vi "generate_smgr.vi"() -> ()   [LabVIEW 2010]
uses:
  lib/Global 2.vi
  <vilib>/measure/NI_MABase.lvlib
  <vilib>/measure/NI_MAPro.lvlib
panel:
  out "file path out":path
  out "Waveform Graph":waveform(i16)[](graph)
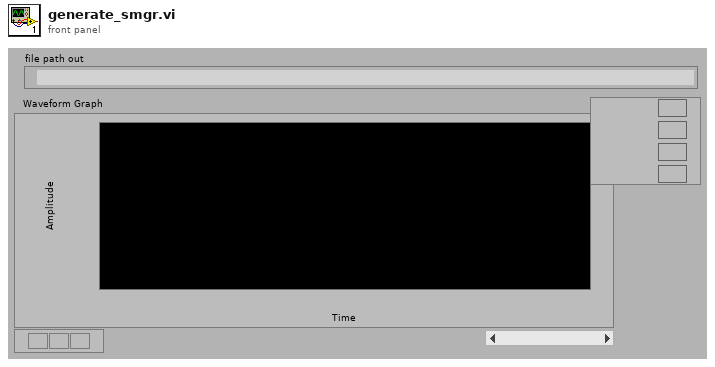
[diagram p1: front panel]
types:
  T1 = cluster{"frequency":dbl, "amplitude":dbl, "phase":dbl}[][]
  T2 = cluster{"actualSamples":i32, "absoluteInitialX":dbl, "relativeInitialX":dbl, "xIncrement":dbl, "offset":dbl, "gain":dbl, "reserved1":dbl, "reserved2":dbl}
  T3 = cluster{"wfm info":cluster{"actualSamples":i32, "absoluteInitialX":dbl, "relativeInitialX":dbl, "xIncrement":dbl, "offset":dbl, "gain":dbl, "reserved1":dbl, "reserved2":dbl}[], "wfm":i16[][]}
  T4 = cluster{"name":enum16{"sync", "phase_a", "phase_b", "phase_c", "ground"}, "num":i32, "Numeric":i32}[]
  T5 = enum16{"sync", "phase_a", "phase_b", "phase_c", "ground"}
  T6 = cluster{"actualSamples":i32, "absoluteInitialX":dbl, "relativeInitialX":dbl, "xIncrement":dbl, "offset":dbl, "gain":dbl, "reserved1":dbl, "reserved2":dbl}[]
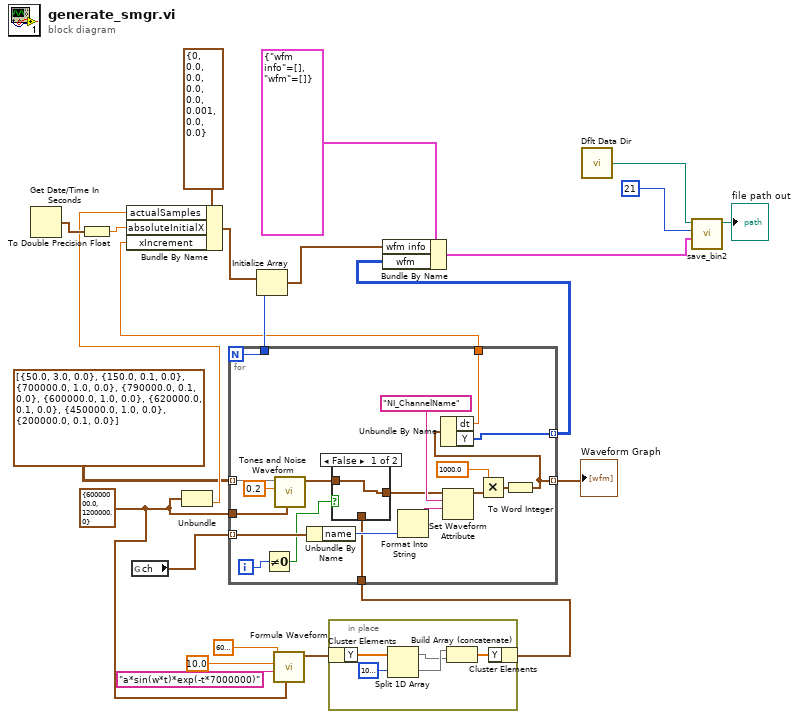
[diagram p0: block diagram]
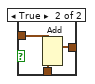
[diagram p2: hidden frame]
diagram:
  w6 = cluster{"Fs":dbl, "#s":dbl} {"Fs"=60000000.0, "#s"=1200000.0} ("sampling info")
  n1 = Get Date/Time In Seconds() -> (seconds since 1Jan1904=w12:timestamp)
  n2 = To Double Precision Float(number=w12) -> (double precision float=w13:dbl)
  n3 = global read "Global 2.vi" "ch"() -> (w18:T4)
  n4 = Unbundle(w6) -> ("#s"=w11:dbl)  [unwired: 1 out]
  n5 = call <vilib>:"Formula Waveform.vi"("sampling info"=w6, "formula"="a*sin(w*t)*exp(-t*7000000)", "amplitude"=10.0, "frequency"=6000000.0) -> ("signal out"=w3:waveform(dbl))  [unwired: 6 in, 1 out]
  n6 = in-place {
    n7 = in-place-cluster #1(w3) -> ("Y"=w25:dbl[])
    n8 = Split 1D Array(array=w25, index=1000000) -> (first subarray=w26:dbl[], second subarray=w27:dbl[])
    n9 = Build Array (concatenate)(w27, w26) -> (w24:dbl[])
    n10 = in-place-cluster #1("Y"=w24) -> (w2:waveform(dbl))
  }
  n11 = for {
    N -> [w43]
    tunnel: w18 -> [w47] mode=indexing
    tunnel: [w31] -> w1 mode=indexing
    tunnel: w6 -> [w40]
    tunnel: [w43] -> w16
    tunnel: [w32] -> w10 mode=indexing
    tunnel: [w41] -> w14
    tunnel: T1 [[{"frequency"=50.0, "amplitude"=3.0, "phase"=0.0}, {"frequency"=150.0, "amplitude"=0.1, "phase"=0.0}], [{"frequency"=700000.0, "amplitude"=1.0, "phase"=0.0}, {"frequency"=790000.0, "amplitude"=0.1, "phase"=0.0}], [{"frequency"=600000.0, "amplitude"=1.0, "phase"=0.0}, {"frequency"=620000.0, "amplitude"=0.1, "phase"=0.0}], [{"frequency"=450000.0, "amplitude"=1.0, "phase"=0.0}, {"frequency"=200000.0, "amplitude"=0.1, "phase"=0.0}]] -> [w39] mode=indexing
    tunnel: w2 -> [w36]
    i -> [w30]
    n12 = Not Equal To 0?(x=w30) -> (x != 0?=w29:bool)
    n13 = call <vilib>:"Tones and Noise Waveform.vi"("sampling info"=w40, "noise (rms)"=0.2, "tones"=w39) -> ("signal out"=w37:waveform(dbl))  [unwired: 7 in, 1 out]
    n14 = Unbundle By Name(w47) -> ("name"=w46:T5)
    n15 = case shown="False" w29 {
      tunnel: w37 -> [w48 w51]
      tunnel: w36 -> [_ w50]
      tunnel: [w48 w49] -> w35
      frame False {
      }
      frame True {
        n16 = Add(1:w50, 2:w51) -> (0:w49:waveform(dbl))  [unwired: 1 in, 1 out]
      }
    }
    n17 = Format Into String(w46) -> (resulting string=w45:string)  [unwired: 3 in, 1 out]
    n18 = Set Waveform Attribute(5:w45, 6:"NI_ChannelName" ("name"), 7:w35) -> (3:w34:waveform(dbl))  [unwired: 1 in, 2 out]
    n19 = Multiply(x=1000.0, y=w34) -> (x*y=w33:waveform(dbl))
    n20 = To Word Integer(number=w33) -> (16bit integer=w31:waveform(i16))
    n21 = Unbundle By Name(w31) -> ("dt"=w41:dbl, "Y"=w32:i16[])
  }
  "Waveform Graph" <- w1
  n22 = Bundle By Name(cluster=T2 {"actualSamples"=0, "absoluteInitialX"=0.0, "relativeInitialX"=0.0, "xIncrement"=0.0, "offset"=0.0, "gain"=0.001, "reserved1"=0.0, "reserved2"=0.0} ("wfm info 2"), "actualSamples"=w11, "absoluteInitialX"=w13, "xIncrement"=w14) -> (w17:T2)
  n23 = Initialize Array(w17, w16) -> (w15:T6)
  n24 = Bundle By Name(cluster=T3 {"wfm info"=[], "wfm"=[]} ("xz"), "wfm info"=w15, "wfm"=w10) -> (w20:T3)
  n25 = call <vilib>:"Dflt Data Dir.vi"() -> ("App:Default Data Directory"=w23:path)
  n26 = call "save_bin2.vi"("xz"=w20, "DevNo"=21, "start path"=w23) -> ("file path out"=→"file path out":path)  [unwired: 2 in, 2 out]
